vi "rad_Add Files to App Image.vi"(8 "error in (no error)":errorcluster, 10 "Files to Add":path[](array[path]), 11 "AppImage Path":path) -> (0 "error out":errorcluster, 3 "AppImage Path":path)   [LabVIEW 2014]
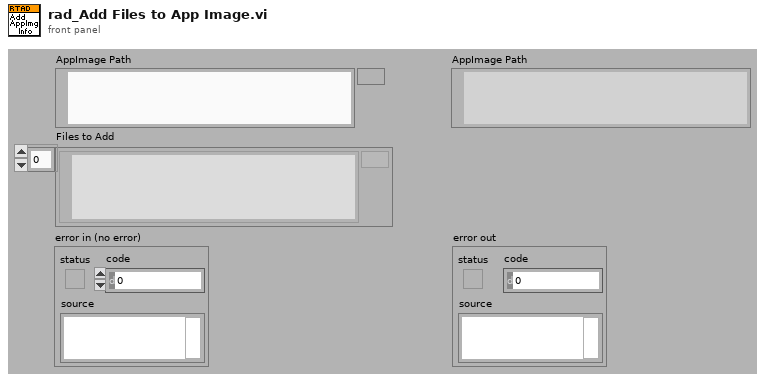
[diagram p1: front panel]
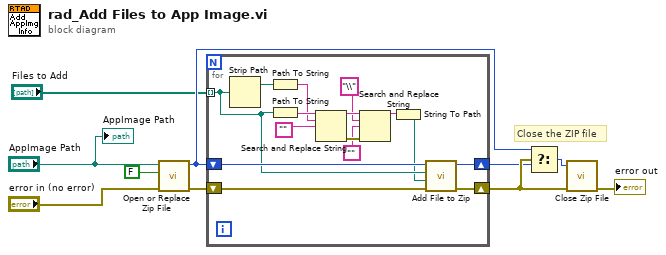
[diagram p0: block diagram]
diagram:
  # "Close the ZIP file"
  n1 = call "Open or Replace Zip File.vi"("error in (no error)"="error in (no error)", "Replace (T) or Open?"=FALSE, "target"="AppImage Path") -> ("error out"=w5:errorcluster, "zip file out"=w4:i64)  [unwired: 2 in, 1 out]
  n2 = for {
    tunnel: "Files to Add" -> [w21] mode=indexing
    shift-right: [w24] -> w8
    shift-left: w4 -> [w22]
    shift-right: [w25] -> w9
    shift-left: w5 -> [w23]
    n3 = Strip Path(path=w21) -> (stripped path=w20:path)  [unwired: 1 out]
    n4 = Path To String(path=w20) -> (string=w18:string)
    n5 = Path To String(path=w21) -> (string=w19:string)
    n6 = Search and Replace String(input string=w19, search string=w18, replace string="") -> (result string=w15:string, error out=w14:errorcluster)  [unwired: 1 in, 6 out]
    n7 = Search and Replace String(input string=w15, search string="\\", replace string="", error in=w14) -> (result string=w11:string)  [unwired: 7 out]
    n8 = String To Path(string=w11) -> (path=w16:path)
    n9 = call <vilib>:"Add File to Zip.vi"("error in (no error)"=w23, "destination path in zip"=w16, "source file path"=w21, "zip file in"=w22) -> ("error out"=w25:errorcluster, "zip file out"=w24:i64)  [unwired: 6 out]
  }
  n10 = Select(t=w4, s=w9, f=w8) -> (s? t:f=w7:i64)
  n11 = call <vilib>:"Close Zip File.vi"("error in (no error)"=w9, "zip file in"=w7) -> ("error out"=→"error out":errorcluster)  [unwired: 1 in, 4 out]
  "AppImage Path" <- "AppImage Path"
